vi "FFT Max 5 Values.vi"(11 "Signals":waveform(dbl)) -> (2 "FFT Overview":cluster{"f0":dbl, "df":dbl, "magnitude":dbl[]}(graph), 3 "Frequency array":cluster{"Amplitude":dbl, "Frequency":dbl}[](array[cluster]))   [LabVIEW 2014, in "Aquisicao de Dados.lvlib"]
uses:
  Aquisicao de Dados.lvlib
  <vilib>/express/express analysis/Spectral/Block/exnSpectralBlock spectral measurements peak poly.vi
  <vilib>/express/express analysis/Spectral/Block/exnSpectralBlock spectral measurements peak WFM.vi
  <vilib>/express/express analysis/Spectral/XNode/ExpressSpectralMeasurementsBlockNode.xnode
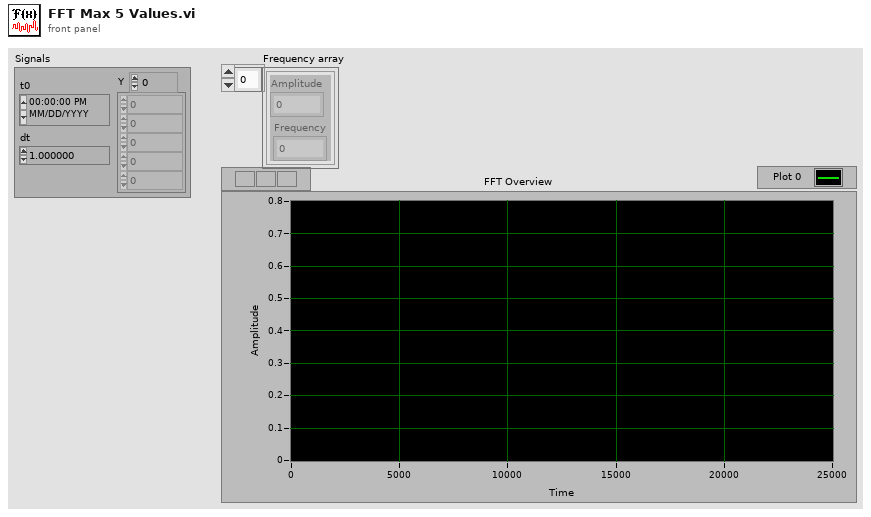
[diagram p1: front panel]
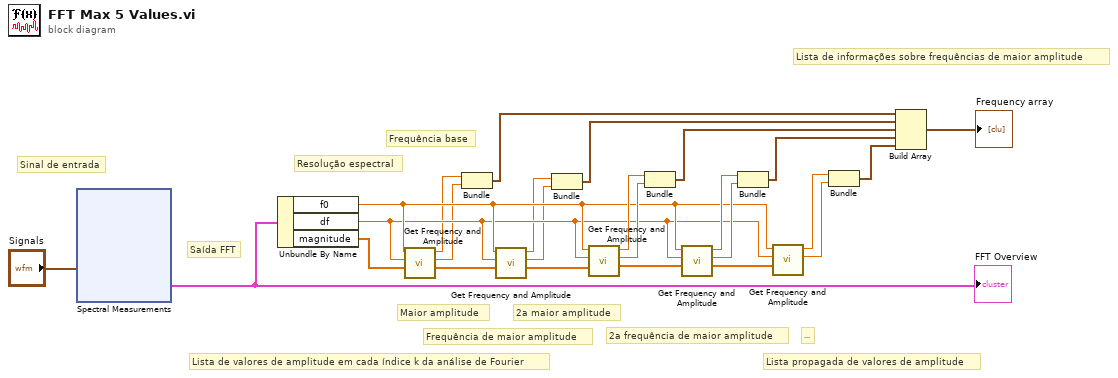
[diagram p0: block diagram]
diagram:
  # "Sinal de entrada"
  # "Lista propagada de valores de amplitude"
  # "Lista de informações sobre frequências de maior amplitude"
  # "..."
  # "2a maior amplitude"
  # "2a frequência de maior amplitude"
  # "Maior amplitude"
  # "Frequência de maior amplitude"
  # "Lista de valores de amplitude em cada índice k da análise de Fourier"
  # "Resolução espectral"
  # "Frequência base"
  # "Saída FFT"
  n1 = xnode "Spectral Measurements"("Signals"="Signals") -> ("FFT - (Peak)"=w2:cluster{"f0":dbl, "df":dbl, "magnitude":dbl[]})  [unwired: 1 in, 2 out]
  "FFT Overview" <- w2
  n2 = Unbundle By Name(w2) -> ("f0"=w13:dbl, "df"=w12:dbl, "magnitude"=w5:dbl[])
  n3 = call "Get Frequency and Amplitude.vi"("Array in"=w5, "df"=w12, "f0"=w13) -> ("Array out"=w8:dbl[], "Frequency"=w7:dbl, "Amplitude"=w6:dbl)  [unwired: 6 in]
  n4 = Bundle("Amplitude"=w6, "Frequency"=w7) -> (w3:cluster{"Amplitude":dbl, "Frequency":dbl})  [unwired: 1 in]
  n5 = call "Get Frequency and Amplitude.vi"("Array in"=w8, "df"=w12, "f0"=w13) -> ("Array out"=w21:dbl[], "Frequency"=w10:dbl, "Amplitude"=w9:dbl)  [unwired: 6 in]
  n6 = Bundle("Amplitude"=w9, "Frequency"=w10) -> (w11:cluster{"Amplitude":dbl, "Frequency":dbl})  [unwired: 1 in]
  n7 = call "Get Frequency and Amplitude.vi"("Array in"=w21, "df"=w12, "f0"=w13) -> ("Array out"=w22:dbl[], "Frequency"=w16:dbl, "Amplitude"=w15:dbl)  [unwired: 6 in]
  n8 = Bundle("Amplitude"=w15, "Frequency"=w16) -> (w14:cluster{"Amplitude":dbl, "Frequency":dbl})  [unwired: 1 in]
  n9 = call "Get Frequency and Amplitude.vi"("Array in"=w22, "df"=w12, "f0"=w13) -> ("Array out"=w23:dbl[], "Frequency"=w18:dbl, "Amplitude"=w17:dbl)  [unwired: 6 in]
  n10 = Bundle("Amplitude"=w17, "Frequency"=w18) -> (w24:cluster{"Amplitude":dbl, "Frequency":dbl})  [unwired: 1 in]
  n11 = call "Get Frequency and Amplitude.vi"("Array in"=w23, "df"=w12, "f0"=w13) -> ("Frequency"=w20:dbl, "Amplitude"=w19:dbl)  [unwired: 6 in, 1 out]
  n12 = Bundle("Amplitude"=w19, "Frequency"=w20) -> (w25:cluster{"Amplitude":dbl, "Frequency":dbl})  [unwired: 1 in]
  n13 = Build Array(w3, w11, w14, w24, w25) -> (→"Frequency array":cluster{"Amplitude":dbl, "Frequency":dbl}[])
